vi "BMark_Get App From Ring Selection.vi"(10 "all projects":T1[](array[typedef]), 11 "Projects":u16) -> (3 "App Info":T1)   [LabVIEW 2013]
uses:
  <vilib>/addons/analyzer/_analyzerctrls.llb/VIAnCtl Analysis App Info.ctl
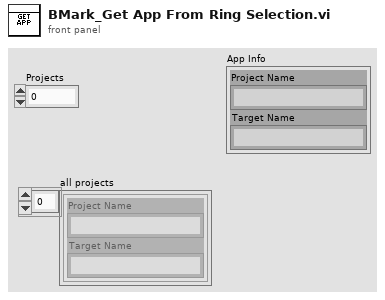
[diagram p1: front panel]
types:
  T1 = typedef "VIAnCtl Analysis App Info.ctl" = cluster{"Project Name":string, "Target Name":string}
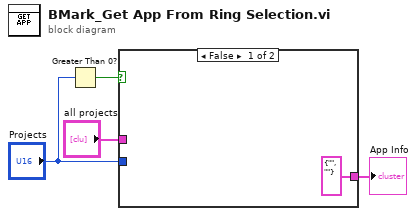
[diagram p0: block diagram]
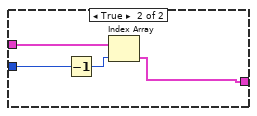
[diagram p2: hidden frame]
diagram:
  n1 = Greater Than 0?(x="Projects") -> (x > 0?=w3:bool)
  n2 = case shown="False" w3 {
    tunnel: "all projects" -> [_ w9]
    tunnel: "Projects" -> [_ w8]
    tunnel: [T1 {"Project Name"="", "Target Name"=""} ("App Info") w6] -> w4
    frame False {
    }
    frame True {
      n3 = Decrement(x=w8) -> (x-1=w7:u16)
      n4 = Index Array(array=w9, index=w7) -> (element=w6:T1)
    }
  }
  "App Info" <- w4
